vi "calc_focus_test.vi"() -> ()   [LabVIEW 2019]
uses:
  <vilib>/vision/NI_Vision_Development_Module.lvlib
  gVision/gVision.lvlib
panel:
  out "focus":sgl
  out "error out":errorcluster
  out "Image":T1(plugin-control)
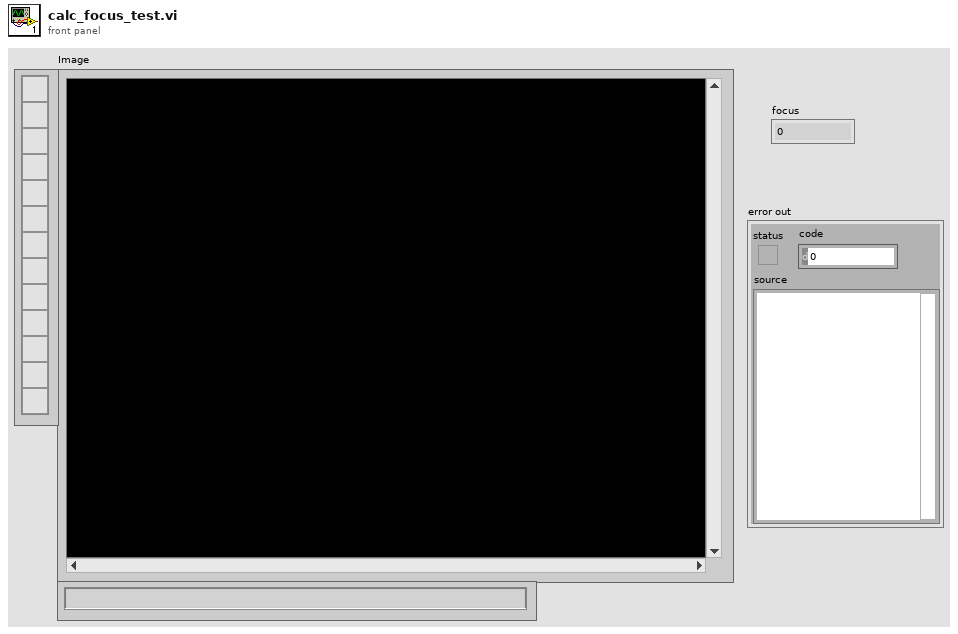
[diagram p1: front panel]
types:
  T1 = typedef "IMAQ Image.ctl" = refnum<image>
  T2 = typedef "Image Type" = u32
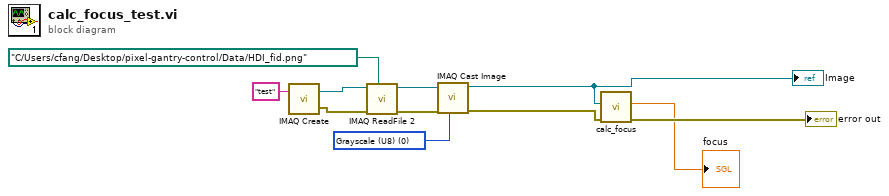
[diagram p0: block diagram]
diagram:
  w5 = T2 0 items=["Grayscale (U8)", "Grayscale (I16)", "Grayscale (SGL)", "Complex (CSG)", "RGB (U32)", "HSL (U32)", "RGB (U64)", "Grayscale (U16)"] ("Image Type")
  n1 = call "IMAQ Create"("Image Name"="test") -> ("New Image"=w11:T1, "error out"=w9:errorcluster)  [unwired: 4 in]
  n2 = call "IMAQ ReadFile 2"("File Path"=path "C:/Users/cfang/Desktop/pixel-gantry-control/Data/HDI_fid.png", "error in (no error)"=w9, "Image"=w11) -> ("error out"=w7:errorcluster, "Image Out"=w6:T1)  [unwired: 4 in, 3 out]
  n3 = call "IMAQ Cast Image"("Image Type"=w5, "error in (no error)"=w7, "Image Src"=w6) -> ("error out"=w3:errorcluster, "Image Dst Out"=w4:T1)  [unwired: 7 in]
  "Image" <- w4
  n4 = call "calc_focus.vi"("error in"=w3, "Image"=w4) -> ("error out"=→"error out":errorcluster, "focus"=→"focus":sgl)  [unwired: 7 in, 1 out]
